vi "Get Component Settings.vi"(8 "error in (no error)":errorcluster, 9 "settings id":T1={"plugin"=-1, "thread"=-1, "group"=-1, "transfer"=-1, "channel"=-1}, 11 "Configuration Session in":refnum<class "Configuration Session.lvclass">) -> (0 "error out":errorcluster, 2 "component settings":T2[](array[typedef]), 3 "Configuration Session out":refnum<class "Configuration Session.lvclass">)   [LabVIEW 2019, in "DSF Core.lvlib" / "Configuration Session.lvclass"]
uses:
  Configuration Session.lvclass
  Typedefs/DSF Settings Info.ctl
  Typedefs/DSF Configuration ID.ctl
  Configuration Session.lvclass/Configuration Session.ctl
  DSF Core.lvlib
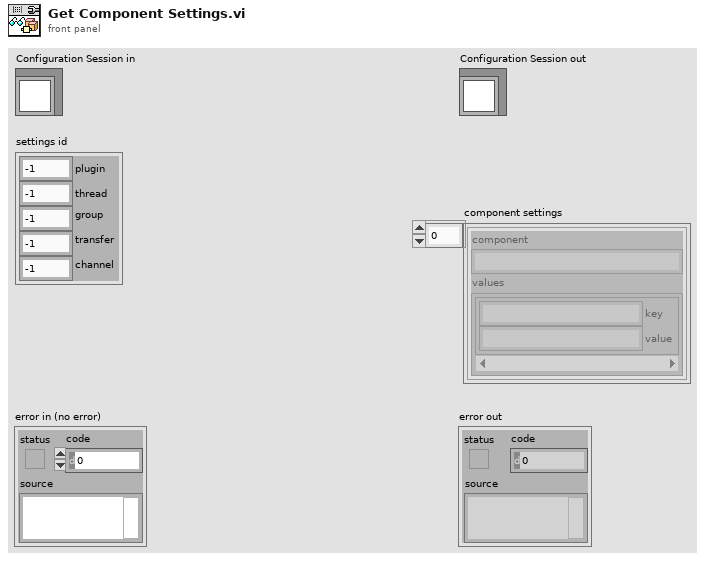
[diagram p1: front panel]
types:
  T1 = typedef "DSF Core.lvlib/DSF Configuration ID.ctl" = cluster{"plugin":i32, "thread":i32, "group":i32, "transfer":i32, "channel":i32}
  T2 = typedef "DSF Core.lvlib/DSF Settings Info.ctl" = cluster{"component":string, "values":cluster{"key":string, "value":string}[]}
  T3 = typedef "DSF Core.lvlib/Configuration Session.lvclass/DSF Config Data Ref.ctl" = refnum<data-value>
  T4 = typedef "DSF Core.lvlib/Configuration Session.lvclass/DSF Config Data.ctl" = cluster{"dsf configuration":T5, "path":path, "dirty":bool}
  T5 = typedef "DSF Core.lvlib/Configuration Session.lvclass/Internal DSF Configuration.ctl" = cluster{"dsfversion":T6, "version":T6, "plugins":T7[], "groups":T21[], "transfers":T23[], "channels":T25[], "settings":T27[], "framework configuration":T29, "configuration":refnum<class>}
  T6 = typedef "DSF Core.lvlib/DSF Version Info.ctl" = cluster{"major":u32, "minor":u32, "fix":u32, "build":string}
  T7 = typedef "DSF Core.lvlib/Configuration Session.lvclass/Internal DSF Plugin with ID.ctl" = cluster{"id":string, "values":T8}
  T8 = typedef "DSF Core.lvlib/Configuration Session.lvclass/Internal DSF Plugin Info.ctl" = cluster{"components":string[], "timing":T9, "group ids":string[], "settings id":string, "threads":T10[]}
  T9 = typedef "DSF Core.lvlib/DSF Timing Info.ctl" = cluster{"priority":u64, "decimation":u64, "offset":u64}
  T10 = typedef "DSF Core.lvlib/DSF Engine Plugin Thread Configuration.ctl" = cluster{"core":T11, "component settings":T2[], "transfer groups":T12[]}
  T11 = typedef "DSF Core.lvlib/Thread Configuration.lvclass/Core Thread Configuration.ctl" = cluster{"processor":i32, "priority offset":i16}
  T12 = typedef "DSF Core.lvlib/DSF Engine Transfer Group Configuration.ctl" = cluster{"core":T13, "component settings":T2[], "transfers":T16[]}
  T13 = typedef "DSF Core.lvlib/Group Configuration.lvclass/Core Group Configuration.ctl" = cluster{"name":string, "direction":T14, "cycle timing":T9, "timeout behavior":T15, "enable conversion":bool}
  T14 = typedef "DSF Core.lvlib/DSF Direction.ctl" = enum8{"Tx", "Rx"}
  T15 = typedef "DSF Core.lvlib/DSF Timeout Behavior.ctl" = enum8{"Increment Late Count", "Throw Error"}
  T16 = typedef "DSF Core.lvlib/DSF Engine Transfer Configuration.ctl" = cluster{"core":T17, "component settings":T2[], "channels":T18[]}
  T17 = typedef "DSF Core.lvlib/Transfer Configuration.lvclass/Core Transfer Configuration.ctl" = cluster{"name":string}
  T18 = typedef "DSF Core.lvlib/DSF Engine Channel Configuration.ctl" = cluster{"core":T19, "component settings":T2[]}
  T19 = typedef "DSF Core.lvlib/Channel Configuration.lvclass/Core Channel Configuration.ctl" = cluster{"name":string, "units":string, "engine data type":T20, "string data type":T20, "string offset":u64}
  T20 = typedef "DSF Core.lvlib/DSF Data Type.ctl" = enum8{"Bool", "SGL", "DBL", "I8", "I16", "I32", "I64", "U8", "U16", "U32", "U64"}
  T21 = typedef "DSF Core.lvlib/Configuration Session.lvclass/Internal DSF Group with ID.ctl" = cluster{"id":string, "values":T22}
  T22 = typedef "DSF Core.lvlib/Configuration Session.lvclass/Internal DSF Group Info.ctl" = cluster{"direction":i32, "timing":T9, "transfer ids":string[], "settings id":string, "thread":i32, "timeout behavior":u8}
  T23 = typedef "DSF Core.lvlib/Configuration Session.lvclass/Internal DSF Transfer with ID.ctl" = cluster{"id":string, "values":T24}
  T24 = typedef "DSF Core.lvlib/Configuration Session.lvclass/Internal DSF Transfer Info.ctl" = cluster{"byte order":i32, "channel ids":string[], "settings id":string}
  T25 = typedef "DSF Core.lvlib/Configuration Session.lvclass/Internal DSF Channel with ID.ctl" = cluster{"id":string, "values":T26}
  T26 = typedef "DSF Core.lvlib/Configuration Session.lvclass/Internal DSF Channel Info.ctl" = cluster{"string buffer offset":u64, "string data type":i32, "engine data type":i32, "settings id":string, "units":string}
  T27 = typedef "DSF Core.lvlib/Configuration Session.lvclass/Internal DSF Settings with ID.ctl" = cluster{"id":string, "values":T28}
  T28 = typedef "DSF Core.lvlib/Configuration Session.lvclass/Internal DSF Settings Info.ctl" = cluster{"key":string, "value":string}[]
  T29 = typedef "DSF Core.lvlib/DSF Engine Framework Configuration.ctl" = cluster{"plugins":T30[]}
  T30 = typedef "DSF Core.lvlib/DSF Engine Plugin Configuration.ctl" = cluster{"core":T31, "component settings":T2[], "threads":T10[]}
  T31 = typedef "DSF Core.lvlib/Plugin Configuration.lvclass/Core Plugin Configuration.ctl" = cluster{"name":string, "components":string[], "cycle timing":T9}
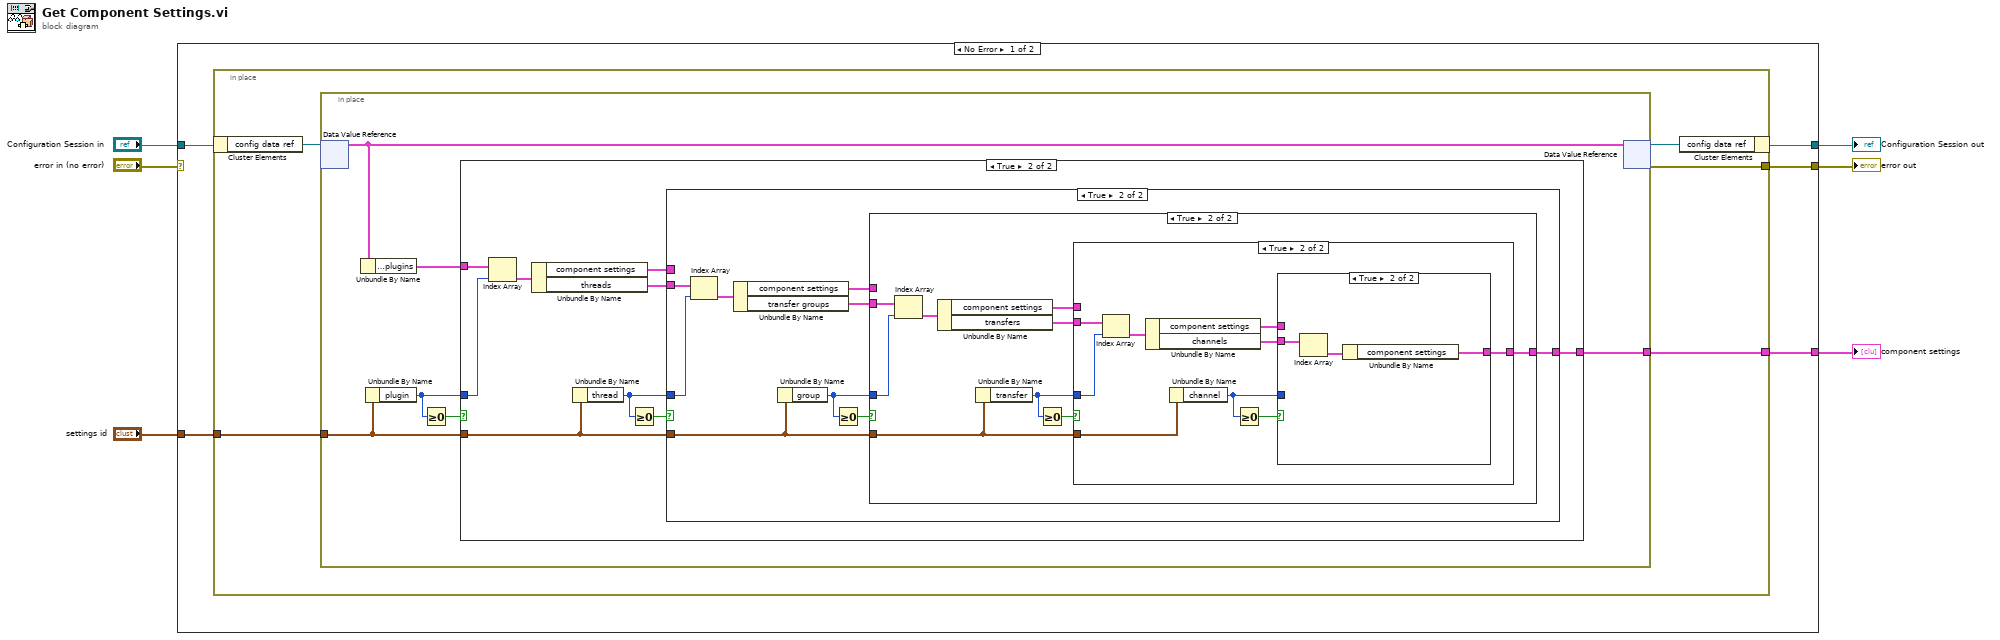
[diagram p0: block diagram]
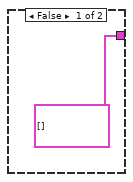
[diagram p2: hidden frame]
diagram:
  n1 = case shown="No Error" "error in (no error)" {
    selector: "error in (no error)" -> [_ w67]
    tunnel: [w8 w68] -> w4
    tunnel: "Configuration Session in" -> [w11 w68]
    tunnel: "settings id" -> [w9 _]
    tunnel: [w10 w67] -> w2
    tunnel: [w7 _] -> w1
    frame No Error {
      n2 = in-place {
        in-place-border: [w15] -> w10
        in-place-border: w9 -> [w14]
        in-place-border: [w12] -> w7
        n3 = in-place-cluster #1(w11) -> ("config data ref"=w16:T3)
        n4 = in-place {
          in-place-border: w14 -> [w20]
          in-place-border: [w21] -> w12
          n5 = in-place-dvr #2(w16) -> (w18:T4)  [unwired: 1 out]
          n6 = Unbundle By Name(w18) -> ("dsf configuration.framework configuration.plugins"=w17:T30[])
          n7 = Unbundle By Name(w20) -> ("plugin"=w19:i32)
          n8 = Greater Or Equal To 0?(x=w19) -> (x >= 0?=w22:bool)
          n9 = case shown="True" w22 {
            tunnel: [T2[] [] ("component settings") w28] -> w21
            tunnel: w20 -> [_ w31]
            tunnel: w19 -> [_ w24]
            tunnel: w17 -> [_ w25]
            frame False {
            }
            frame True {
              n10 = Index Array(array=w25, index=w24) -> (element=w27:T30)
              n11 = Unbundle By Name(w27) -> ("component settings"=w29:T2[], "threads"=w26:T10[])
              n12 = Unbundle By Name(w31) -> ("thread"=w30:i32)
              n13 = Greater Or Equal To 0?(x=w30) -> (x >= 0?=w32:bool)
              n14 = case shown="True" w32 {
                tunnel: w31 -> [_ w42]
                tunnel: w30 -> [_ w35]
                tunnel: w29 -> [w33 _]
                tunnel: [w33 w36] -> w28
                tunnel: w26 -> [_ w38]
                frame False {
                }
                frame True {
                  n15 = Index Array(array=w38, index=w35) -> (element=w39:T10)
                  n16 = Unbundle By Name(w39) -> ("component settings"=w37:T2[], "transfer groups"=w34:T12[])
                  n17 = Unbundle By Name(w42) -> ("group"=w40:i32)
                  n18 = Greater Or Equal To 0?(x=w40) -> (x >= 0?=w41:bool)
                  n19 = case shown="True" w41 {
                    tunnel: w42 -> [_ w52]
                    tunnel: w40 -> [_ w47]
                    tunnel: w37 -> [w43 _]
                    tunnel: [w43 w44] -> w36
                    tunnel: w34 -> [_ w48]
                    frame False {
                    }
                    frame True {
                      n20 = Index Array(array=w48, index=w47) -> (element=w49:T12)
                      n21 = Unbundle By Name(w49) -> ("component settings"=w45:T2[], "transfers"=w46:T16[])
                      n22 = Unbundle By Name(w52) -> ("transfer"=w50:i32)
                      n23 = Greater Or Equal To 0?(x=w50) -> (x >= 0?=w51:bool)
                      n24 = case shown="True" w51 {
                        tunnel: w52 -> [_ w62]
                        tunnel: w50 -> [_ w57]
                        tunnel: w46 -> [_ w58]
                        tunnel: w45 -> [w53 _]
                        tunnel: [w53 w54] -> w44
                        frame False {
                        }
                        frame True {
                          n25 = Index Array(array=w58, index=w57) -> (element=w59:T16)
                          n26 = Unbundle By Name(w59) -> ("component settings"=w55:T2[], "channels"=w56:T18[])
                          n27 = Unbundle By Name(w62) -> ("channel"=w60:i32)
                          n28 = Greater Or Equal To 0?(x=w60) -> (x >= 0?=w61:bool)
                          n29 = case shown="True" w61 {
                            tunnel: w60 -> [_ _]
                            tunnel: w56 -> [_ w65]
                            tunnel: w55 -> [w63 _]
                            tunnel: [w63 w64] -> w54
                            frame False {
                            }
                            frame True {
                              n30 = Index Array(array=w65) -> (element=w66:T18)  [unwired: 1 in]
                              n31 = Unbundle By Name(w66) -> ("component settings"=w64:T2[])
                            }
                          }
                        }
                      }
                    }
                  }
                }
              }
            }
          }
          n32 = in-place-dvr #2(w18) -> (w13:T3, w15:errorcluster)
        }
        n33 = in-place-cluster #1("config data ref"=w13) -> (w8:refnum<class "Configuration Session.lvclass">)
      }
    }
    frame Error {
    }
  }
  "error out" <- w2
  "Configuration Session out" <- w4
  "component settings" <- w1
